vi "Mouse_Over.vi"(10 "Bounds":T2[](array[typedef]), 11 "Refs cluster In":T1) -> (1 "Onto":bool[](array[boolean]), 3 "Refs cluster Out":T1)   [LabVIEW 2015]
uses:
  <vilib>/Utility/miscctls.llb/LVRectTypeDef.ctl
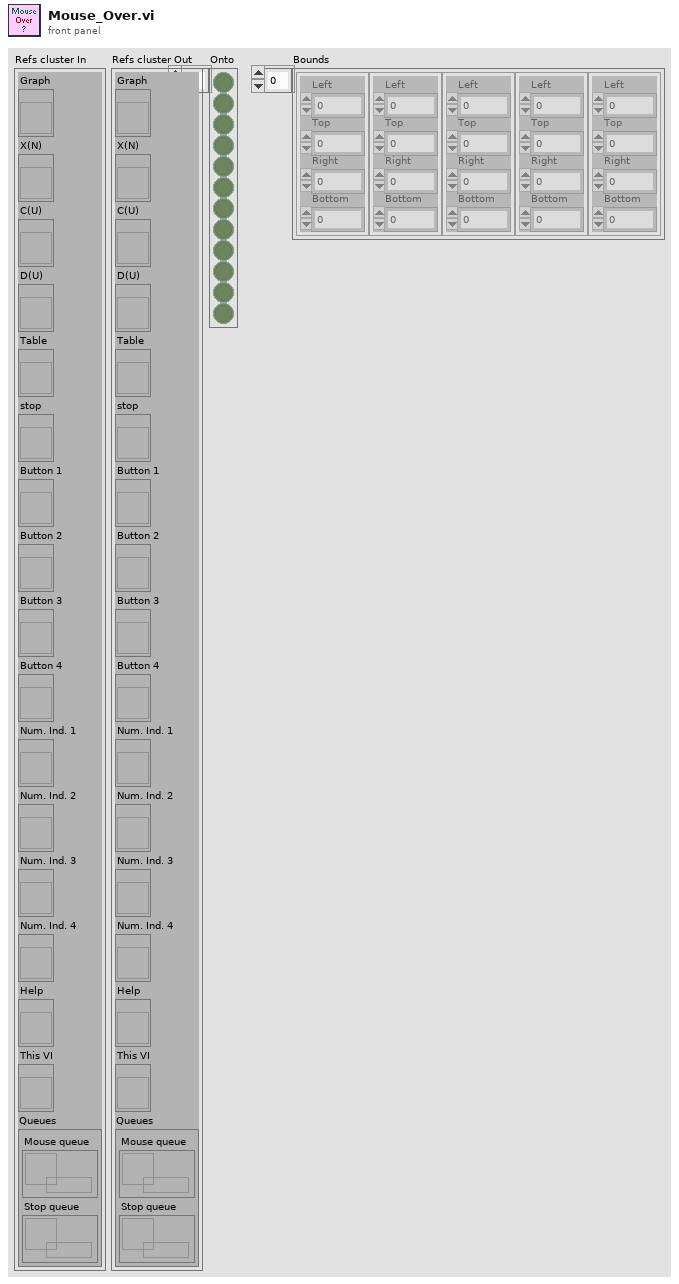
[diagram p1: front panel]
types:
  T1 = cluster{"Graph":refnum<vi>, "X(N)":refnum<vi>, "C(U)":refnum<vi>, "D(U)":refnum<vi>, "Table":refnum<vi>, "stop":refnum<vi>, "Button 1":refnum<vi>, "Button 2":refnum<vi>, "Button 3":refnum<vi>, "Button 4":refnum<vi>, "Num. Ind. 1":refnum<vi>, "Num. Ind. 2":refnum<vi>, "Num. Ind. 3":refnum<vi>, "Num. Ind. 4":refnum<vi>, "Help":refnum<vi>, "This VI":refnum<vi>, "Queues":cluster{"Mouse queue":refnum<queue>, "Stop queue":refnum<queue>}}
  T2 = typedef "LVRectTypeDef.ctl" = cluster{"Left":i16, "Top":i16, "Right":i16, "Bottom":i16}
  T3 = cluster{"device ID":refnum<k1>, "axis info":cluster{"Horizontal":i32, "Vertical":i32, "Scrolling":i32}, "button info":cluster{"button 1":bool, "button 2":bool, "button 3":bool, "button 4":bool}}
  T4 = cluster{"Horizontal":i32, "Vertical":i32, "Scrolling":i32}
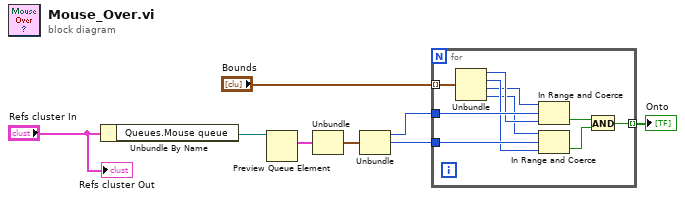
[diagram p0: block diagram]
diagram:
  n1 = Unbundle By Name("Refs cluster In") -> ("Queues.Mouse queue"=w2:refnum<queue>)
  n2 = Preview Queue Element(queue=w2) -> (element=w7:T3)  [unwired: 2 in, 3 out]
  n3 = Unbundle(w7) -> ("axis info"=w6:T4)  [unwired: 2 out]
  n4 = Unbundle(w6) -> ("Horizontal"=w5:i32, "Vertical"=w4:i32)  [unwired: 1 out]
  n5 = for {
    tunnel: "Bounds" -> [w18] mode=indexing
    tunnel: w5 -> [w17]
    tunnel: w4 -> [w16]
    tunnel: [w9] -> w3 mode=indexing
    n6 = Unbundle(w18) -> ("Left"=w15:i16, "Top"=w14:i16, "Right"=w13:i16, "Bottom"=w12:i16)
    n7 = In Range and Coerce(upper limit=w13, x=w17, lower limit=w15) -> (In Range?=w11:bool)  [unwired: 1 out]
    n8 = In Range and Coerce(upper limit=w12, x=w16, lower limit=w14) -> (In Range?=w10:bool)  [unwired: 1 out]
    n9 = And(x=w11, y=w10) -> (x .and. y?=w9:bool)
  }
  "Onto" <- w3
  "Refs cluster Out" <- "Refs cluster In"
